vi "Stop Core.vi"(10 "final error code":i32, 11 "Chamber Controller in":refnum<class "Chamber Controller.lvclass">) -> (3 "Chamber Controller out":refnum<class "Chamber Controller.lvclass">)   [LabVIEW 2020, in "Chamber Controller.lvlib" / "Chamber Controller.lvclass"]
doc: "(<B>Filename</B>: Actor Framework.lvlib:Actor.lvclass:Stop Core.vi)\n\nDefines what the actor does before it stops. Use the <B>final error code</B> input to determine whether the actor shut down in response to an error.\n\nBy default, this method passes the Stop message along to all auto-stop nested actors. A descendant class may override this method to define additional behavior, such as shutting down any processes the actor initiated in its override of the Actor Core method."
uses:
  Chamber Controller.lvclass
  Chamber Controller.lvclass/Chamber Controller.ctl
  <vilib>/MGI/Monitored Actor/Monitored Actor/Monitored Actor/Monitored Actor.lvclass
  _Abstract Classes/Abstract Chamber/Abstract Chamber.lvclass
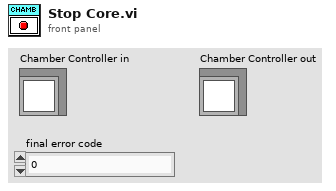
[diagram p1: front panel]
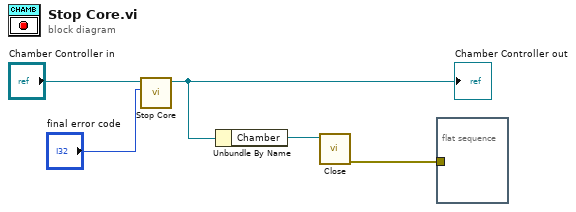
[diagram p0: block diagram]
diagram:
  n1 = call-parent "Stop Core.vi"("final error code"="final error code", "Monitored Actor in"="Chamber Controller in") -> ("Monitored Actor out"=w3:refnum<class "Chamber Controller.lvclass">)  [unwired: 9 in]
  "Chamber Controller out" <- w3
  n2 = Unbundle By Name(w3) -> ("Chamber"=w2:refnum<class "Abstract Chamber.lvclass">)
  n3 = call-dynamic "Close.vi"("Chamber in"=w2) -> ("error out"=w1:errorcluster)  [unwired: 9 in, 1 out]
  n4 = flat-sequence {
    tunnel: w1 -> [_]
    frame #0 {
    }
  }
